vi "SetParam.vi"(8 "error in (no error)":errorcluster caption="entrée d'erreur (pas d'erreur)", 10 "KBinsDiscretizer":T1={"n_bins"=[5], "encode"="onehot", "strategy"="quantile"}, 11 "KBinsDiscretizer.lvclass":refnum<class "KBinsDiscretizer.lvclass">) -> (0 "error out":errorcluster caption="sortie d'erreur", 3 "KBinsDiscretizer.lvclass":refnum<class "KBinsDiscretizer.lvclass">)   [LabVIEW 2020, in "KBinsDiscretizer.lvclass"]
doc: "Set Parameters"
uses:
  KBinsDiscretizer.lvclass
  KBinsDiscretizer.lvclass/KBinsDiscretizer.ctl
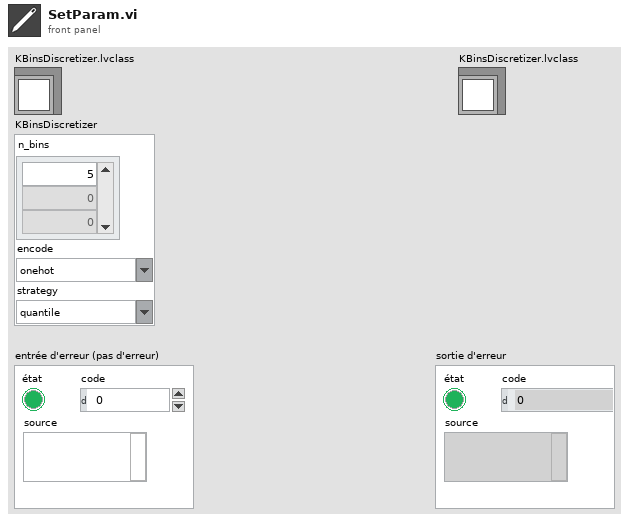
[diagram p1: front panel]
types:
  T1 = cluster{"n_bins":i32[], "encode":string, "strategy":string}
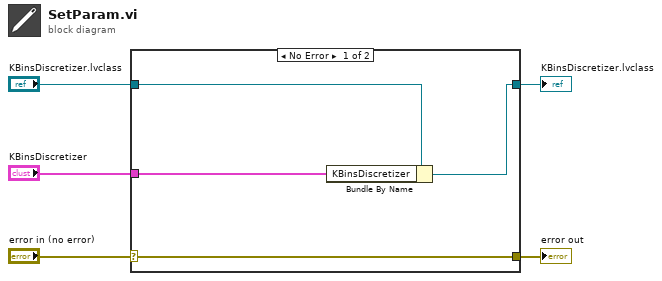
[diagram p0: block diagram]
diagram:
  n1 = case shown="No Error" "error in (no error)" {
    selector: "error in (no error)" -> [w9 w10]
    tunnel: [w9 w10] -> w4
    tunnel: [w7 w11] -> w2
    tunnel: "KBinsDiscretizer.lvclass" -> [w8 w11]
    tunnel: "KBinsDiscretizer" -> [w6 _]
    frame No Error {
      n2 = Bundle By Name(cluster=w8, "KBinsDiscretizer"=w6) -> (w7:refnum<class "KBinsDiscretizer.lvclass">)
    }
    frame Error {
    }
  }
  "error out" <- w4
  "KBinsDiscretizer.lvclass" <- w2
